vi "Throw Error - Queue Already Exists.vi"(8 "Error In":errorcluster, 11 "Queue Name":string) -> (0 "Error Out":errorcluster)   [LabVIEW 2023, in "Error Manager.lvlib"]
doc: "Issues a command to the Process module by enqueuing into the Process module queue."
uses:
  Error Manager.lvlib
panel:
  # "Input\nInputs to the VI"
  # "Development\nControls or indicators that are useful for development or testing, but which are not outputs of the VI."
  # "Output\nOutputs of the VI"
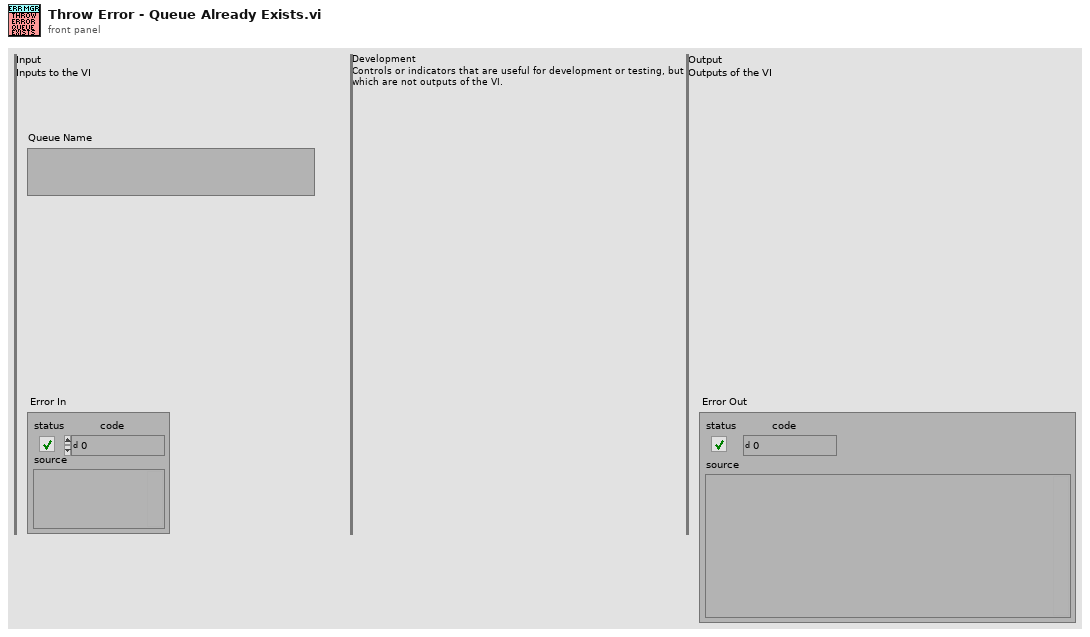
[diagram p1: front panel]
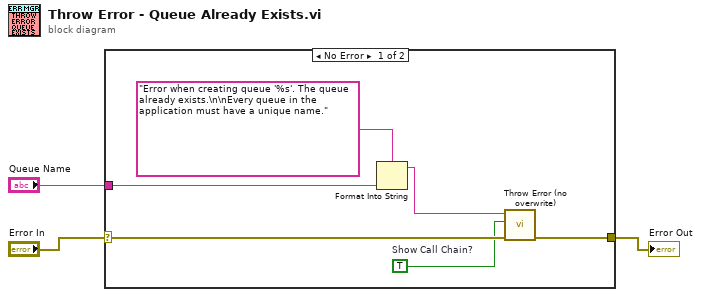
[diagram p0: block diagram]
diagram:
  n1 = case shown="No Error" "Error In" {
    selector: "Error In" -> [w9 w10]
    tunnel: [w8 w10] -> w2
    tunnel: "Queue Name" -> [w5 _]
    frame No Error {
      w4 = TRUE  # Show Call Chain?
      n2 = Format Into String(format string="Error when creating queue '%s'. The queue already exists.\n\nEvery queue in the application must have a unique name.", w5) -> (resulting string=w7:string)  [unwired: 2 in, 1 out]
      n3 = call "Throw Error (no overwrite).vi"(8:w9, 10:w4, 11:w7) -> (0:w8:errorcluster)  [unwired: 8 in]
    }
    frame Error {
      # "If error at input, do not overwrite."
    }
  }
  "Error Out" <- w2
